vi "Configure Series.vi"(6 "Series CFG":string, 8 "error in (no error)":errorcluster, 9 "Virt Instrs CFG":string, 10 "Instr CFGs":string[](array[string]), 11 "HAL GOOP4:Series Base in":refnum<class "Series Base.lvclass">) -> (0 "error out":errorcluster, 3 "HAL GOOP4:Series Base out":refnum<class "Series Base.lvclass">)   [LabVIEW 2023, in "HAL GOOP4.lvlib" / "Series Base.lvclass"]
uses:
  Series Base.lvclass
  Series Base.lvclass/Series Base.ctl
  <vilib>/JDP Science/JSONtext/Next JSON Value.vi
  <vilib>/JDP Science/JSONtext/String Subset.vi
  <vilib>/JDP Science/JSONtext/Parsing/Advance past next JSON Value (inlined COPY).vi
  <vilib>/JDP Science/JSONtext/Parsing/Advance past whitespace.vi
  <vilib>/JDP Science/JSONtext/Parsing/Advance past String.vi
  <vilib>/JDP Science/JSONtext/Parsing/Advance past Number.vi
  <vilib>/JDP Science/JSONtext/Parsing/Advance past Line Ending.vi
  <vilib>/JDP Science/JSONtext/Parsing/Parse Full Path or Item Name.vi
  <vilib>/JDP Science/JSONtext/Parsing/Advance past Array.vi
  <vilib>/JDP Science/JSONtext/Parsing/Advance past Object.vi
  <vilib>/JDP Science/JSONtext/support/Error Cluster From Code.vi
  <vilib>/JDP Science/JSONtext/Offset/Find Item Locations by Path.vi
  <vilib>/Utility/error.llb/Error Cluster From Error Code.vi
  <vilib>/JDP Science/JSONtext/support/Format JSON Array Text.vi
  <vilib>/ErrorRing/Error Ring.xnode
  <vilib>/JDP Science/JSONtext/JSONtext.lvlib
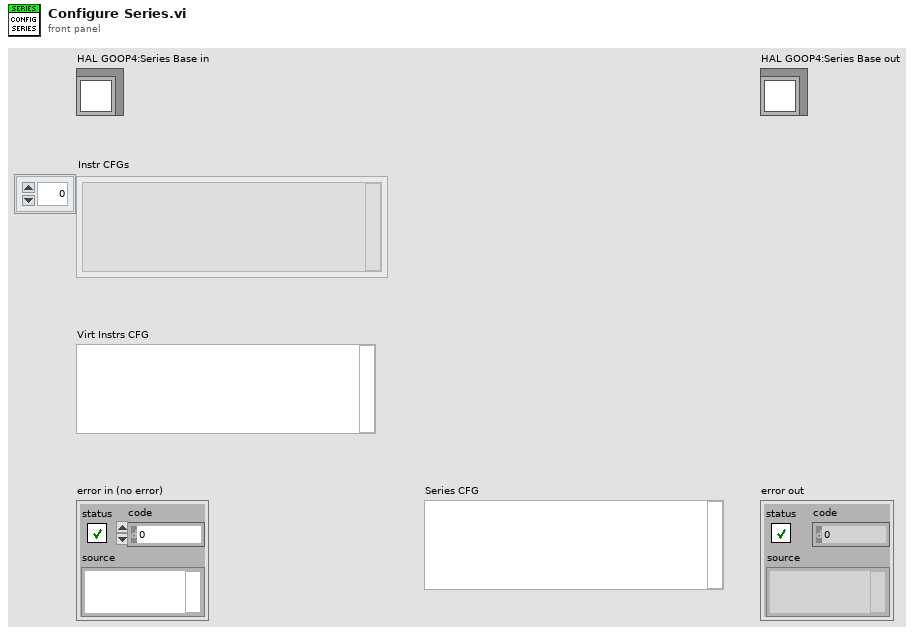
[diagram p1: front panel]
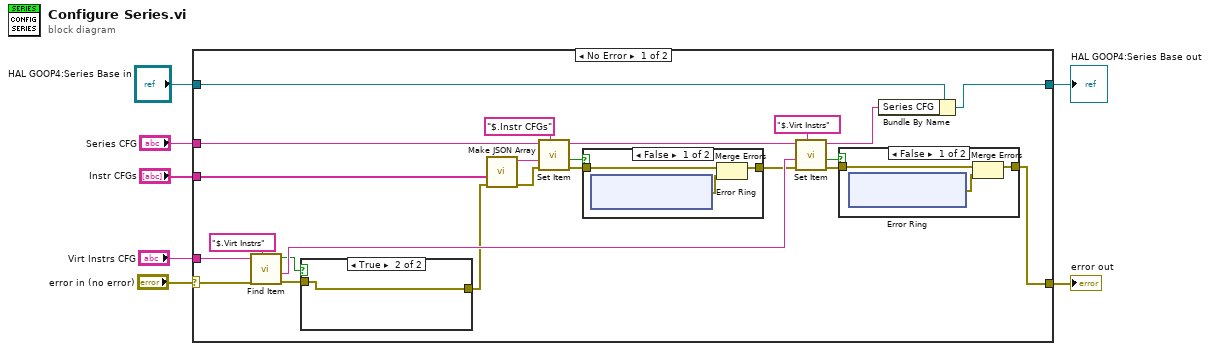
[diagram p0: block diagram]
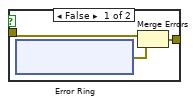
[diagram p4: hidden frame]
diagram:
  n1 = case shown="No Error" "error in (no error)" {
    selector: "error in (no error)" -> [w19 w58]
    tunnel: [w8 w58] -> w6
    tunnel: [w29 w59] -> w4
    tunnel: "HAL GOOP4:Series Base in" -> [w30 w59]
    tunnel: "Virt Instrs CFG" -> [w18 _]
    tunnel: "Series CFG" -> [w23 _]
    tunnel: "Instr CFGs" -> [w26 _]
    frame No Error {
      n2 = call <vilib>:"Find Item.vi"("$Path or Item Name"="$.Virt Instrs", "error in (no error)"=w19, "JSON"=w18) -> ("error out"=w14:errorcluster, "<JSON>"=w16:string, "Found"=w15:bool)  [unwired: 5 in, 1 out]
      n3 = case shown="True" w15 {
        tunnel: w14 -> [w51 w57]
        tunnel: [w49 w57] -> w13
        frame False {
          n4 = xnode "Error Ring"() -> ("error out"=w50:errorcluster)
          n5 = Merge Errors(w51, w50) -> (w49:errorcluster)
        }
        frame True {
        }
      }
      n6 = call <vilib>:"Make JSON Array.vi"("error in (no error)"=w13, "JSON Elements"=w26) -> ("error out"=w22:errorcluster, "<JSON>"=w25:string)  [unwired: 8 in]
      n7 = call <vilib>:"Set Item.vi"("$Path or Item Name"="$.Instr CFGs", "error in (no error)"=w22, "JSON to Insert"=w25, "JSON"=w23) -> ("error out"=w21:errorcluster, "Replaced"=w11:bool, "<JSON>"=w20:string)  [unwired: 4 in]
      n8 = case shown="False" w11 {
        tunnel: w21 -> [w42 w48]
        tunnel: [w41 w48] -> w12
        frame False {
          n9 = xnode "Error Ring"() -> ("error out"=w40:errorcluster)
          n10 = Merge Errors(w42, w40) -> (w41:errorcluster)
        }
        frame True {
        }
      }
      n11 = call <vilib>:"Set Item.vi"("$Path or Item Name"="$.Virt Instrs", "error in (no error)"=w12, "JSON to Insert"=w16, "JSON"=w20) -> ("error out"=w9:errorcluster, "Replaced"=w10:bool, "<JSON>"=w27:string)  [unwired: 4 in]
      n12 = case shown="False" w10 {
        tunnel: w9 -> [w33 w39]
        tunnel: [w32 w39] -> w8
        frame False {
          n13 = xnode "Error Ring"() -> ("error out"=w31:errorcluster)
          n14 = Merge Errors(w33, w31) -> (w32:errorcluster)
        }
        frame True {
        }
      }
      n15 = Bundle By Name(cluster=w30, "Series CFG"=w27) -> (w29:refnum<class "Series Base.lvclass">)
    }
    frame Error {
    }
  }
  "error out" <- w6
  "HAL GOOP4:Series Base out" <- w4
